vi "MALT GetServiceStatus.vi"(8 "error in":errorcluster, 11 "ServiceName":string) -> (0 "error out":errorcluster, 2 "Status":T1=1 items=["Stopped"=1, "StartPending"=2, "StopPending"=3, "Running"=4, "ContinuePending"=5, "PausePending"=6, "Paused"=7], 3 "FindIt":bool)   [LabVIEW 2018, in "AltonTech MALT200817.lvlib"]
uses:
  AltonTech MALT200817.lvlib
  System.ServiceProcess
  Public/Types/MALT ServiceControlerStatusType.ctl
panel:
  out "Services":string[](array[string])
  in  "reference":refnum<k24>
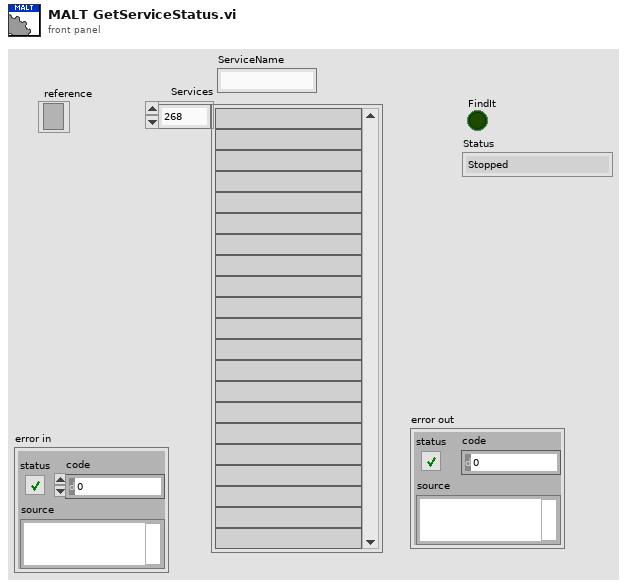
[diagram p1: front panel]
types:
  T1 = typedef "AltonTech MALT200817.lvlib/MALT ServiceControlerStatusType.ctl" = i32
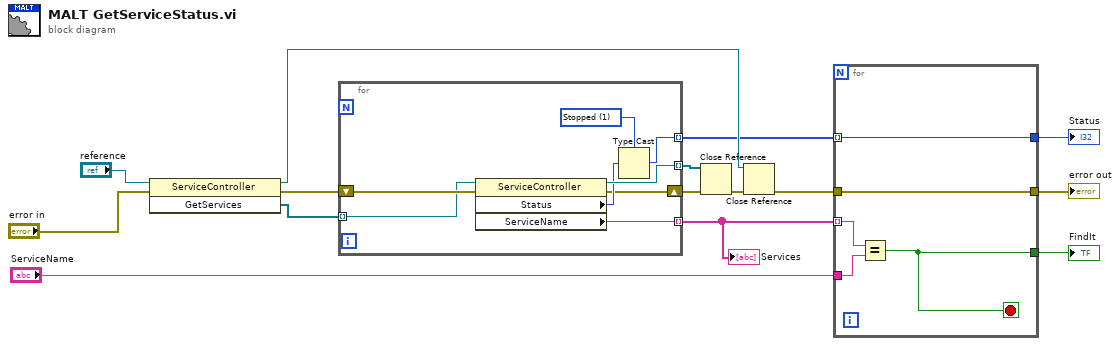
[diagram p0: block diagram]
diagram:
  n1 = invoke on="Invoke Node" class="ServiceController" method="GetServices"(reference="reference", error in="error in") -> (reference out=w9:refnum<k24>, error out=w12:errorcluster, "GetServices"=w15:refnum<k24>[])  [unwired: 1 in]
  n2 = for {
    tunnel: w15 -> [w17] mode=indexing
    tunnel: [w23] -> w14 mode=indexing
    tunnel: [w22] -> w7 mode=indexing
    tunnel: [w20] -> w4 mode=indexing
    shift-right: [w18] -> w11
    shift-left: w12 -> [w19]
    w16 = T1 1 items=["Stopped"=1, "StartPending"=2, "StopPending"=3, "Running"=4, "ContinuePending"=5, "PausePending"=6, "Paused"=7] ("Status")
    n3 = property class="ServiceController"(reference=w17, error in=w19) -> (reference out=w23:refnum<k24>, error out=w18:errorcluster, "Status"=w21:i32, "ServiceName"=w22:string)
    n4 = Type Cast(type=w16, x=w21) -> (*(type *) &x=w20:T1)
  }
  "Services" <- w7
  n5 = Close Reference(reference=w14, error in (no error)=w11) -> (error out=w10:errorcluster)
  n6 = Close Reference(reference=w9, error in (no error)=w10) -> (error out=w1:errorcluster)
  n7 = for {
    tunnel: w7 -> [w28] mode=indexing
    tunnel: "ServiceName" -> [w27]
    tunnel: [w26] -> w5
    tunnel: w4 -> [w25] mode=indexing
    tunnel: [w25] -> w3
    tunnel: [w24] -> w2
    tunnel: w1 -> [w24]
    stop <- w26 stop-if-true
    n8 = Equal?(x=w28, y=w27) -> (x = y?=w26:bool)
  }
  "FindIt" <- w5
  "Status" <- w3
  "error out" <- w2
